vi "Set External Trigger Mode.vi"(8 "error in (no error)":errorcluster, 10 "External Trigger Mode":T1, 11 "hdl":i32) -> (0 "error out":errorcluster, 3 "hdl out":i32)   [LabVIEW 2013, in "Thorlabs_SC10.lvlib"]
uses:
  <instrlib>/Thorlabs_SC10/Thorlabs_SC10.lvlib
  <instrlib>/Thorlabs_SC10/Public/Configure/External Trigger Mode.ctl
  <instrlib>/Thorlabs_SC10/Data/SC10CommandLib_x64.dll
  <instrlib>/Thorlabs_SC10/Data/SC10CommandLib_win32.dll
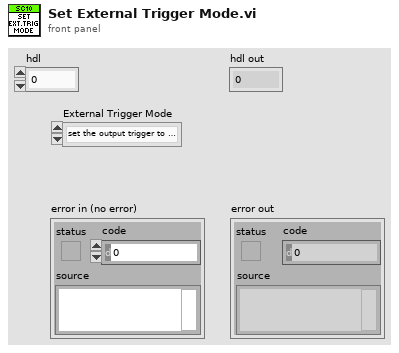
[diagram p1: front panel]
types:
  T1 = typedef "Thorlabs_SC10.lvlib/External Trigger Mode.ctl" = enum16{"set the output trigger to follow the shutter output when the SH05 is connected", "force the trigger output to follow the controller output when an SH05 is equipped"}
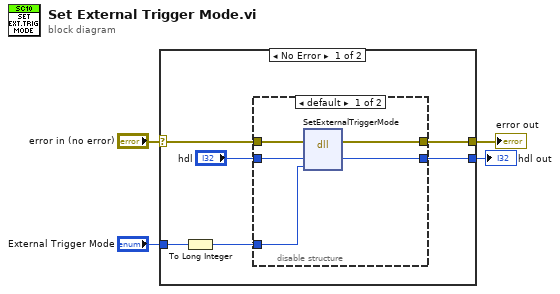
[diagram p0: block diagram]
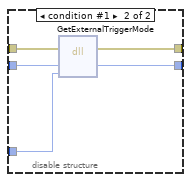
[diagram p2: hidden frame]
diagram:
  n1 = case shown="No Error" "error in (no error)" {
    selector: "error in (no error)" -> [w10 w21]
    tunnel: [w9 w21] -> w4
    tunnel: "External Trigger Mode" -> [w8 _]
    tunnel: [w6 _] -> w1
    frame No Error {
      n2 = To Long Integer(number=w8) -> (32bit integer=w5:i32)
      n3 = disable-structure shown="default" {
        disable-tunnel: w10 -> [w15 w20]
        disable-tunnel: [w14 w19] -> w9
        disable-tunnel: w5 -> [w13 w18]
        disable-tunnel: "hdl" -> [w12 w17]
        disable-tunnel: [w11 w16] -> w6
        frame condition #0 (active) {
          n4 = dll-call lib="C:/Program Files (x86)/National Instruments/LabVIEW 2013/instr.lib/Thorlabs_SC10/Data/SC10CommandLib_win32.dll" fn="SetExternalTriggerMode"(error in=w15, "hdl"=w12, "value"=w13) -> (error out=w14:errorcluster, "hdl"=w11:i32)  [unwired: 4 in, 1 out]
        }
        frame condition #1 {
          n5 = dll-call lib="C:/Program Files/National Instruments/LabVIEW 2013/instr.lib/Thorlabs_SC10/Data/SC10CommandLib_x64.dll" fn="GetExternalTriggerMode"(error in=w20, "hdl"=w17, "value"=w18) -> (error out=w19:errorcluster, "hdl"=w16:i32)  [unwired: 4 in, 1 out]
        }
      }
    }
    frame Error {
    }
  }
  "error out" <- w4
  "hdl out" <- w1
